vi "Call Virtual Instrument.vi"(0 "Vi Call Location":path, 5 "error in (no error)":errorcluster, 6 "Open Front Panel Window":bool, 7 "Wait for end of Execucion":bool, 8 "Run Vi":bool, 9 "Close Panel when Finished":bool) -> (19 "error out":errorcluster)   [LabVIEW 2011]
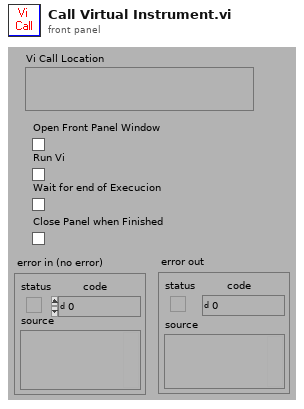
[diagram p1: front panel]
types:
  T1 = enum32{"Bad", "Idle", "Run top level", "Running"}
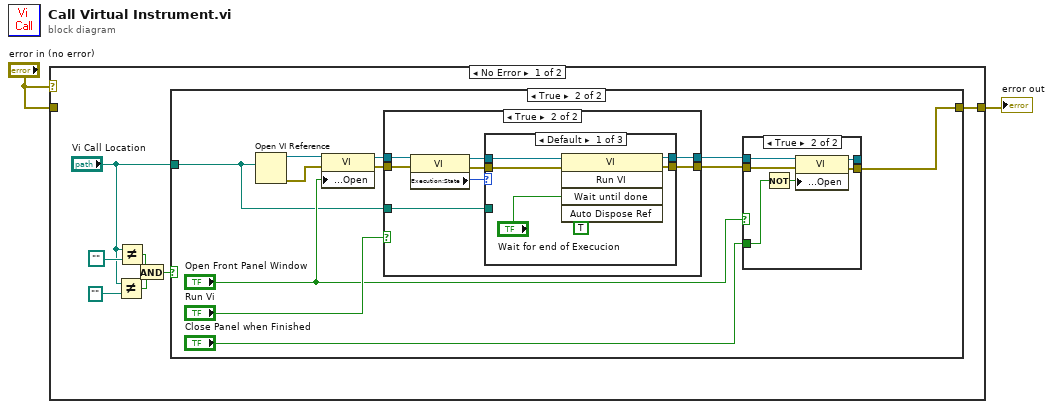
[diagram p0: block diagram]
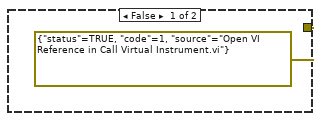
[diagram p2: hidden frame]
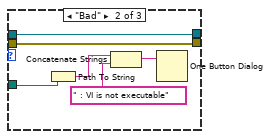
[diagram p5: hidden frame]
diagram:
  n1 = case shown="No Error" "error in (no error)" {
    tunnel: "error in (no error)" -> [_ w54]
    tunnel: [w4 w54] -> w1
    frame No Error {
      n2 = Not Equal?(x="Vi Call Location", y=path "") -> (x != y?=w8:bool)
      n3 = Not Equal?(x="Vi Call Location", y=path "") -> (x != y?=w9:bool)
      n4 = And(x=w9, y=w8) -> (x .and. y?=w3:bool)
      n5 = case shown="True" w3 {
        tunnel: "Vi Call Location" -> [_ w12]
        tunnel: [errorcluster {"status"=TRUE, "code"=1, "source"="Open VI Reference in Call Virtual Instrument.vi"} ("error out") w11] -> w4
        frame False {
        }
        frame True {
          n6 = Open VI Reference(vi path=w12) -> (vi reference=w21:refnum<vi>, error out=w20:errorcluster)  [unwired: 5 in]
          n7 = property class="VI"(reference=w21, error in=w20, "Front Panel Window:Open"="Open Front Panel Window") -> (reference out=w14:refnum<vi>, error out=w19:errorcluster)
          n8 = case shown="True" "Run Vi" {
            tunnel: w14 -> [w31 w37]
            tunnel: w19 -> [w30 w36]
            tunnel: [w31 w39] -> w17
            tunnel: [w30 w38] -> w16
            tunnel: w12 -> [_ w32]
            frame False {
            }
            frame True {
              n9 = property class="VI"(reference=w37, error in=w36) -> (reference out=w34:refnum<vi>, error out=w35:errorcluster, "Execution:State"=w33:T1)
              n10 = case shown="Default" w33 {
                tunnel: [w44 w51 w53] -> w39
                tunnel: [w43 w50 w52] -> w38
                tunnel: w35 -> [w42 w50 w52]
                tunnel: w34 -> [w41 w51 w53]
                tunnel: w32 -> [_ w47 _]
                frame Default {
                  n11 = invoke class="VI" method="Run VI"(reference=w41, error in=w42, "Wait until done"="Wait for end of Execucion", "Auto Dispose Ref"=TRUE ("Auto Dispose Reference")) -> (reference out=w44:refnum<vi>, error out=w43:errorcluster)  [unwired: 1 in, 3 out]
                }
                frame "Bad" {
                  n12 = Path To String(path=w47) -> (string=w46:string)
                  n13 = Concatenate Strings(w46, " : VI is not executable") -> (w48:string)
                  n14 = One Button Dialog(message=w48) -> ()  [unwired: 1 in, 1 out]
                }
                frame "Run top level" {
                }
              }
            }
          }
          n15 = case shown="True" "Open Front Panel Window" {
            tunnel: w17 -> [w23 w29]
            tunnel: w16 -> [w22 w28]
            tunnel: "Close Panel when Finished" -> [_ w27]
            tunnel: [w23 w25] -> _
            tunnel: [w22 w24] -> w11
            frame False {
            }
            frame True {
              n16 = Not(x=w27) -> (.not. x?=w26:bool)
              n17 = property class="VI"(reference=w29, error in=w28, "Front Panel Window:Open"=w26) -> (reference out=w25:refnum<vi>, error out=w24:errorcluster)
            }
          }
        }
      }
    }
    frame Error {
    }
  }
  "error out" <- w1
